vi "RSZVB Set Virtual Transform Ground Loop.vi"(5 "Parameter Type (0)":i32(ring) items=["Capacitance", "Inductance", "Resistance"], 6 "Ground Loop Value (1.0e-12)":dbl=1e-12 format="%^.3e", 7 "Circuit Model (1)":i32(ring)=1 items=["Shunt L"=1, "Shunt C"=2], 8 "error in (no error)":errorcluster {"code" format="%.0x"}, 9 "Function Type (0)":i32(ring) items=["Deembedding", "Embedding"], 10 "Channel (1)":i32=1, 11 "VISA session":refnum<visa-resource-name>) -> (0 "error out":errorcluster {"code" format="%.0x"}, 3 "dup VISA session":refnum<visa-resource-name>)   [LabVIEW 2011]
doc: "This VI specifies the capacitance C, inductance L or resistance R value in the different circuit models for ground loop deembedding/embedding.\n\nRemote-control command(s):\nCALCulate<Ch>:TRANsform:VNETworks:GLOop:DEEMbedding:PARameters:C SC, <capacitance>\nCALCulate<Ch>:TRANsform:VNETworks:GLOop:DEEMbedding:PARameters:L SL, <inductance>\nCALCulate<Ch>:TRANsform:VNETworks:GLOop:DEEMbedding:PARameters:R SC | SL, <resistance>\nCALCulate<Ch>:TRANsform:VNETworks:GLOop:EMBedding:PARameters:C SC,<capacitance>\nCALCulate<Ch>:TRANsform:VNETworks:GLOop:EMBedding:PARameters:L SL, <inductance> \nCALCulate<Ch>:TRANsform:VNETworks:GLOop:EMBedding:PARameters:R SC | SL,<resistance>"
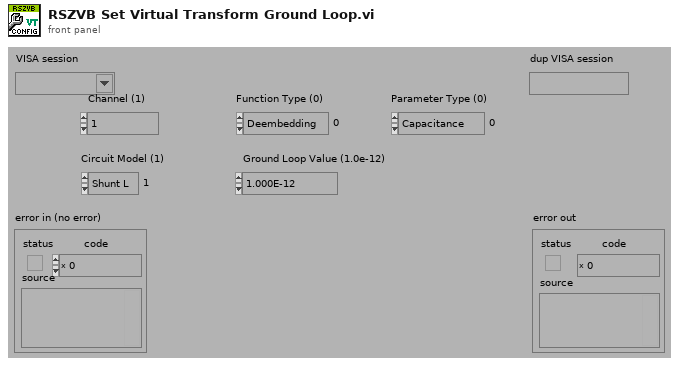
[diagram p1: front panel]
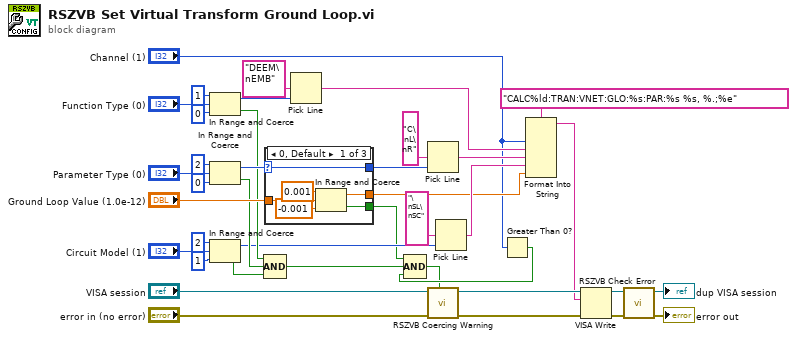
[diagram p0: block diagram]
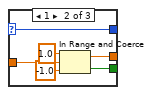
[diagram p2: hidden frame]
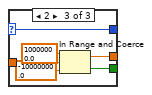
[diagram p3: hidden frame]
diagram:
  n1 = In Range and Coerce(upper limit=1, x="Function Type (0)", lower limit=0) -> (coerced(x)=w22:i32, In Range?=w15:bool)
  n2 = In Range and Coerce(upper limit=2, x="Parameter Type (0)", lower limit=0) -> (coerced(x)=w20:i32, In Range?=w16:bool)
  n3 = In Range and Coerce(upper limit=2, x="Circuit Model (1)", lower limit=1) -> (coerced(x)=w11:i32, In Range?=w17:bool)
  n4 = Compound Arithmetic op=AND(w15, w16, w17) -> (w6:bool)
  n5 = case shown="0, Default" w20 {
    selector: w20 -> [w40 w46 w52]
    tunnel: "Ground Loop Value (1.0e-12)" -> [w45 w51 w57]
    tunnel: [w41 w48 w53] -> w5
    tunnel: [w42 w47 w54] -> w9
    tunnel: [w40 w46 w52] -> w18
    frame 0, Default {
      n6 = In Range and Coerce(upper limit=0.001, x=w45, lower limit=-0.001) -> (coerced(x)=w42:dbl, In Range?=w41:bool)
    }
    frame 1 {
      n7 = In Range and Coerce(upper limit=1.0, x=w51, lower limit=-1.0) -> (coerced(x)=w47:dbl, In Range?=w48:bool)
    }
    frame 2 {
      n8 = In Range and Coerce(upper limit=10000000.0, x=w57, lower limit=-10000000.0) -> (coerced(x)=w54:dbl, In Range?=w53:bool)
    }
  }
  n9 = Pick Line(multi-line string="DEEM\nEMB", line index=w22) -> (output string=w14:string)  [unwired: 1 in]
  n10 = Pick Line(multi-line string="C\nL\nR", line index=w18) -> (output string=w13:string)  [unwired: 1 in]
  n11 = Pick Line(multi-line string="\nSL\nSC", line index=w11) -> (output string=w10:string)  [unwired: 1 in]
  n12 = Greater Than 0?(x="Channel (1)") -> (x > 0?=w4:bool)
  n13 = Compound Arithmetic op=AND(w5, w6, w4) -> (w3:bool)
  n14 = call "RSZVB Coercing Warning.vi"("In Range?"=w3, "error in (no error)"="error in (no error)", "VISA session"="VISA session") -> ("error out"=w35:errorcluster, "dup VISA session"=w36:refnum<visa-resource-name>)  [unwired: 7 in]
  n15 = Format Into String(format string="CALC%ld:TRAN:VNET:GLO:%s:PAR:%s %s, %.;%e", "Channel (1)", w14, w13, w10, w9) -> (resulting string=w7:string)  [unwired: 2 in, 1 out]
  n16 = VISA Write(VISA resource name=w36, write buffer=w7, error in (no error)=w35) -> (VISA resource name out=w39:refnum<visa-resource-name>, error out=w38:errorcluster)  [unwired: 1 out]
  n17 = call "RSZVB Check Error.vi"("error in (no error)"=w38, "VISA session"=w39) -> ("error out"=→"error out":errorcluster, "dup VISA session"=→"dup VISA session":refnum<visa-resource-name>)  [unwired: 8 in]
